vi "Begin.vi"() -> (0 "error out":errorcluster)   [LabVIEW 2018]
doc: "Called before other user functions, this VI is expected to open initial I/O refnums, load in file data, and do all program initialization. Notice that the <B>error out</B> terminal is simply used for data flow. Wiring it to other structures or subVIs ensures that this VI runs first."
uses:
  <vilib>/Rock Robotics/WPI/DriverStation/WPI_DriverStationRobotMode2.ctl
  TypeDefs/typedef_enum_Begin.ctl
  Robot Global Data.vi
  <vilib>/Rock Robotics/Network Tables/NT Write String Array.vi
panel:
  in  "error in":errorcluster
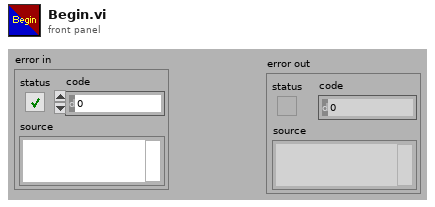
[diagram p1: front panel]
types:
  T1 = typedef "typedef_enum_Begin.ctl" = enum16{"Wrist", "LineFollow", "Gyro", "Climb", "Intake", "Arm", "Drive", "Joysticks"}
  T2 = typedef "WPI_DriverStationRobotMode2.ctl" = enum16{"Autonomous Disabled", "Autonomous Enabled", "Teleop Disabled", "Teleop Enabled", "Disconnected", "Finish", "Test Disabled", "Test Enabled", "Emergency Stopped"}
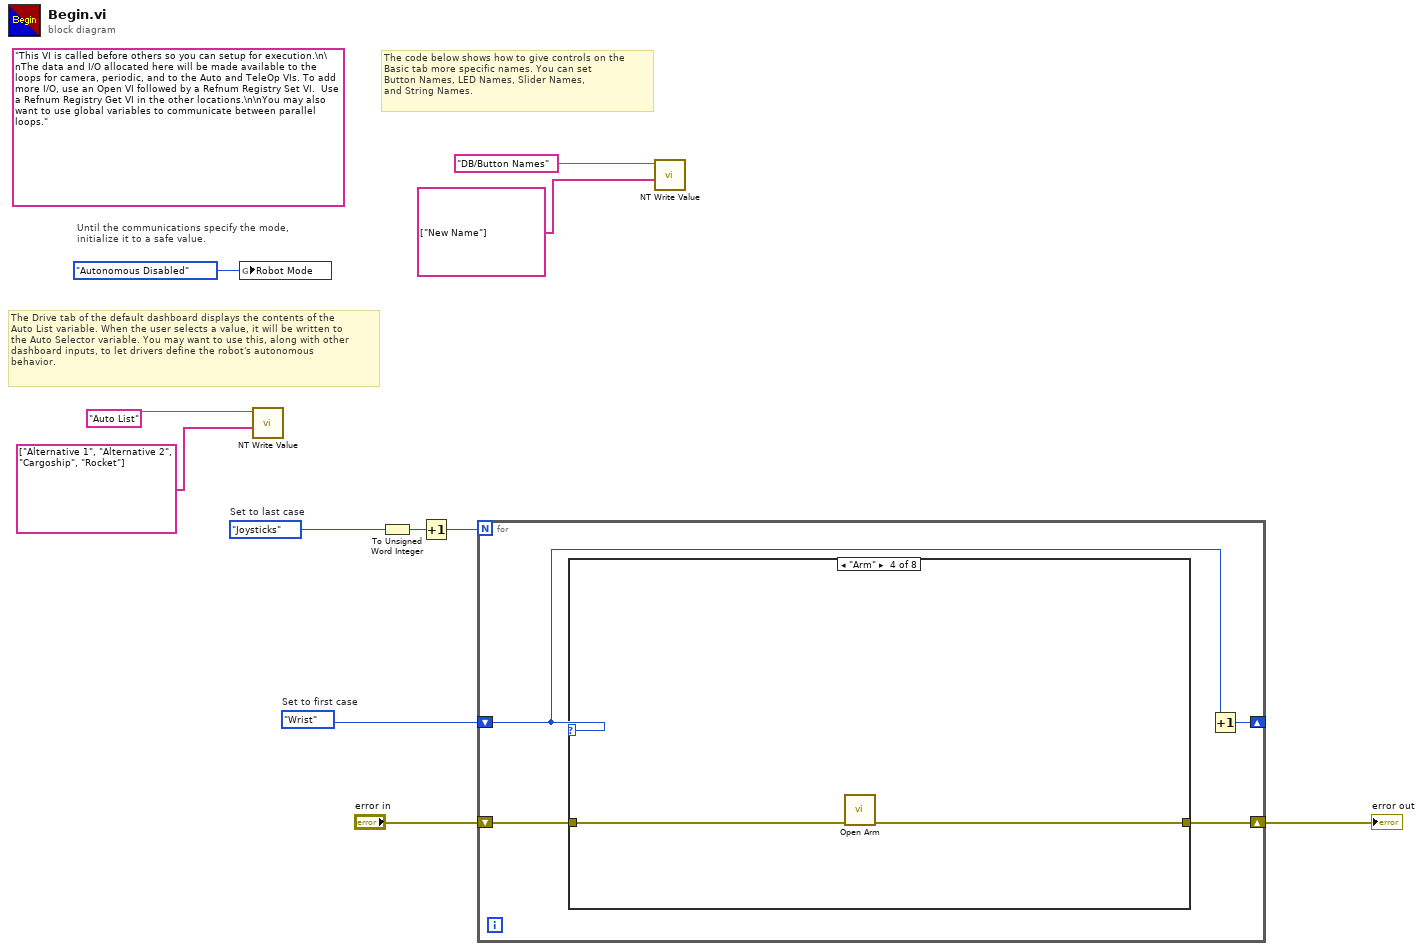
[diagram p0: block diagram]
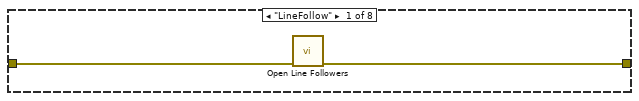
[diagram p2: hidden frame]
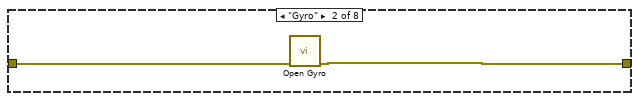
[diagram p3: hidden frame]
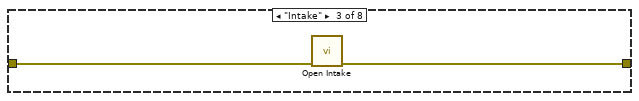
[diagram p4: hidden frame]
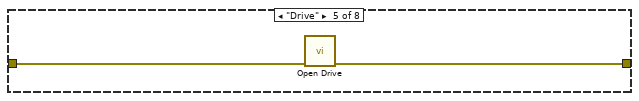
[diagram p5: hidden frame]
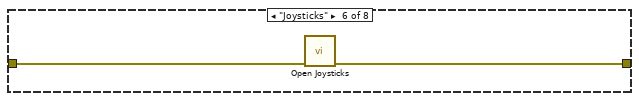
[diagram p6: hidden frame]
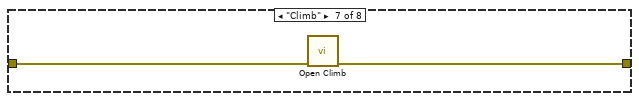
[diagram p7: hidden frame]
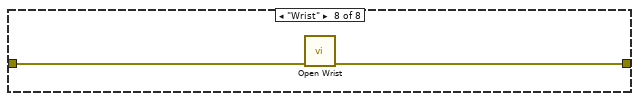
[diagram p8: hidden frame]
diagram:
  w1 = typedef_enum_Begin."Joysticks"  # Set to last case
  w2 = typedef_enum_Begin."Wrist"  # Set to first case
  (unwired) "This VI is called before others so you can setup for execution.\n\nThe data and I/O allocated here will be made available to the loops for camera, periodic, and to the Auto and TeleOp VIs. To add more I/O, use an Open VI followed by a Refnum Registry Set VI.  Use a Refnum Registry Get VI in the other locations.\n\nYou may also want to use global variables to communicate between parallel loops."
  # "The Drive tab of the default dashboard displays the contents of the\nAuto List variable. When the user selects a value, it will be written to\nthe Auto Selector variable. You may want to use this, along with other\ndashboard inputs, to let drivers define the robot's autonomous\nbehavior."
  # "The code below shows how to give controls on the\nBasic tab more specific names. You can set\nButton Names, LED Names, Slider Names,\nand String Names."
  # "Until the communications specify the mode,\ninitialize it to a safe value."
  n1 = global write "Robot Global Data.vi" "Robot Mode"(WPI_DriverStationRobotMode2."Autonomous Disabled" ("Robot Mode")) -> ()
  n2 = call-poly <vilib>:"NT Write Value.vi"("String Array"=string[] ["Alternative 1", "Alternative 2", "Cargoship", "Rocket"], "Name"="Auto List") -> ()  [unwired: 9 in, 1 out]
  n3 = To Unsigned Word Integer(number=w1) -> (unsigned 16bit integer=w6:u16)
  n4 = Increment(x=w6) -> (x+1=w5:u16)
  n5 = for {
    N: w5 -> [_]
    shift-right: [w15] -> _
    shift-left: w2 -> [w14]
    shift-right: [w12] -> w3
    shift-left: "error in" -> [w13]
    n6 = case shown="\"Arm\"" w14 {
      tunnel: w13 -> [w17 w18 w21 w23 w25 w27 w29 w31]
      tunnel: [w16 w19 w20 w22 w24 w26 w28 w30] -> w12
      frame "LineFollow" {
        n7 = call "Open Line Followers.vi"("error in"=w17) -> ("error out"=w16:errorcluster)  [unwired: 10 in]
      }
      frame "Gyro" {
        n8 = call "Open Gyro.vi"("error in (no error)"=w18) -> ("error out"=w19:errorcluster)  [unwired: 10 in]
      }
      frame "Intake" {
        n9 = call "Open Intake.vi"("error in (no error)"=w21) -> ("error out"=w20:errorcluster)  [unwired: 10 in]
      }
      frame "Arm" {
        n10 = call "Open Arm.vi"("error in (no error)"=w23) -> ("error out 2"=w22:errorcluster)  [unwired: 10 in]
      }
      frame "Drive" {
        n11 = call "Open Drive.vi"("error in (no error)"=w25) -> ("error out"=w24:errorcluster)  [unwired: 10 in]
      }
      frame "Joysticks" {
        n12 = call "Open Joysticks.vi"("error in (no error)"=w27) -> ("error out"=w26:errorcluster)  [unwired: 10 in]
      }
      frame "Climb" {
        n13 = call "Open Climb.vi"("error in"=w29) -> ("error out"=w28:errorcluster)  [unwired: 10 in]
      }
      frame "Wrist" {
        n14 = call "Open Wrist.vi"("error in (no error)"=w31) -> ("error out"=w30:errorcluster)  [unwired: 10 in]
      }
    }
    n15 = Increment(x=w14) -> (x+1=w15:T1)
  }
  "error out" <- w3
  n16 = call-poly <vilib>:"NT Write Value.vi"("String Array"=string[] ["New Name"], "Name"="DB/Button Names") -> ()  [unwired: 9 in, 1 out]
